vi "Read LibReader.lvclass.vi"(8 "error in (no error)":errorcluster, 11 "SalProcess in":refnum<class "SalProcess.lvclass">) -> (0 "error out":errorcluster, 2 "LibReader.lvclass":refnum<class "LibReader.lvclass">, 3 "SalProcess out":refnum<class "SalProcess.lvclass">)   [LabVIEW 2018, in "SalProcess.lvclass"]
doc: "Read the LibReader."
uses:
  SalProcess.lvclass
  LibReader/LibReader.lvclass
  SalProcess.lvclass/SalProcess.ctl
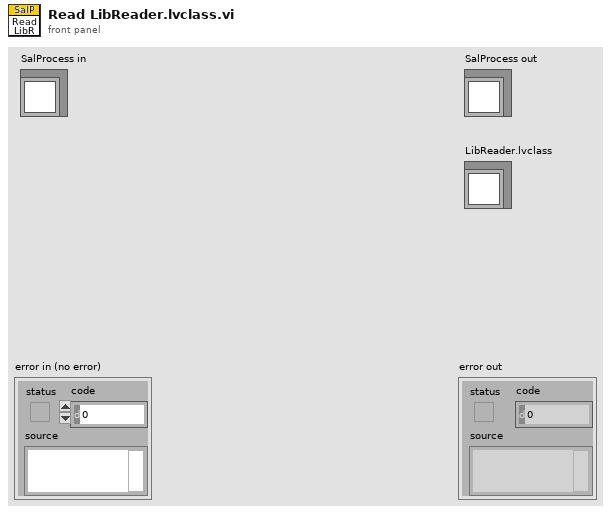
[diagram p1: front panel]
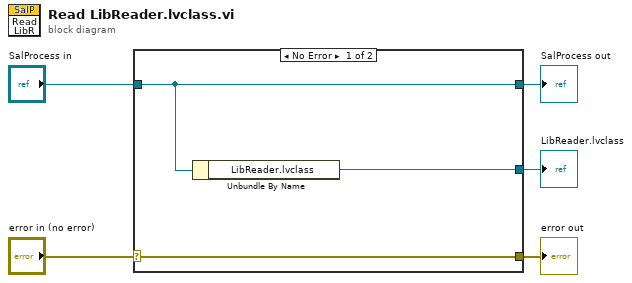
[diagram p0: block diagram]
diagram:
  n1 = case shown="No Error" "error in (no error)" {
    selector: "error in (no error)" -> [w8 w9]
    tunnel: [w8 w9] -> w4
    tunnel: [w7 w10] -> w2
    tunnel: "SalProcess in" -> [w7 w10]
    tunnel: [w6 _] -> w1
    frame No Error {
      n2 = Unbundle By Name(w7) -> ("LibReader.lvclass"=w6:refnum<class "LibReader.lvclass">)
    }
    frame Error {
    }
  }
  "error out" <- w4
  "SalProcess out" <- w2
  "LibReader.lvclass" <- w1
